vi "Initialize With IDN.vi"(0 "VISA resource name":refnum<visa-resource-name>="GPIB0::16::INSTR", 9 "Serial Configuration":T1={"Baud Rate (9600)"=19200, "Flow Control (1: XON/XOFF)"=1, "Termination Char (0:CR)"=0} {"Termination Char (0:CR)" items=["CR", "LF"]; "Flow Control (1: XON/XOFF)" items=["None", "XON/XOFF", "RTS/CTS (2701 Only)", "XON/XOFF & RTS/CTS (2701 Only)"]; "Baud Rate (9600)" items=["300"=300, "600"=600, "1200"=1200, "2400"=2400, "4800"=4800, "9600"=9600, "19.2k"=19200, "38.4k (2701 Only)"=38400, "57.6k (2701 Only)"=57600, "115.2k (2701 Only)"=115200]}, 11 "error in (no error)":errorcluster) -> (4 "VISA resource name out":refnum<visa-resource-name>, 6 "ID Query read buffer":string, 15 "error out":errorcluster)   [LabVIEW 2015]
doc: "This VI opens a VISA session for the VISA resource name specified. You can optionally reset the instrument by setting the front panel reset control. You must run this VI before using any of the instrument driver VIs for this instrument.\n\nNotes:\n\n(1) This instrument driver supports serial communication. If problems are encountered when using serial communication, it is recommended to try using baud rates less than 19,200 and hardware handshaking. \n\n(2) If you do wish to use the serial interface, set the serial settings on the instrument to be the same as the serial settings on the block diagram and in Measurement & Automation Explorer.\n\n(3) This VI sets the instrument to *RST conditions as listed in the manual. This does not include clearing the buffer."
uses:
  <instrlib>/Keithley 27XX/Keithley 27XX.lvlib
panel:
  # "© 2005 National Instruments Corporation.  ALL RIGHTS RESERVED."
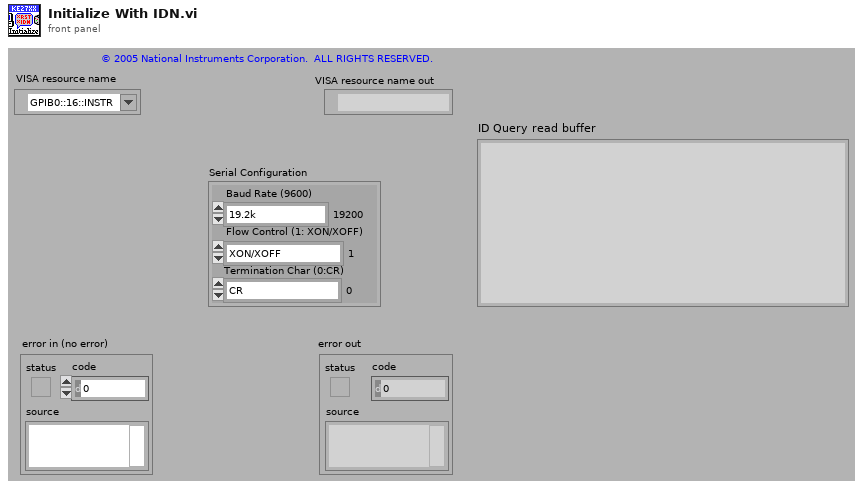
[diagram p1: front panel]
types:
  T1 = cluster{"Baud Rate (9600)":u32, "Flow Control (1: XON/XOFF)":u16, "Termination Char (0:CR)":u16}
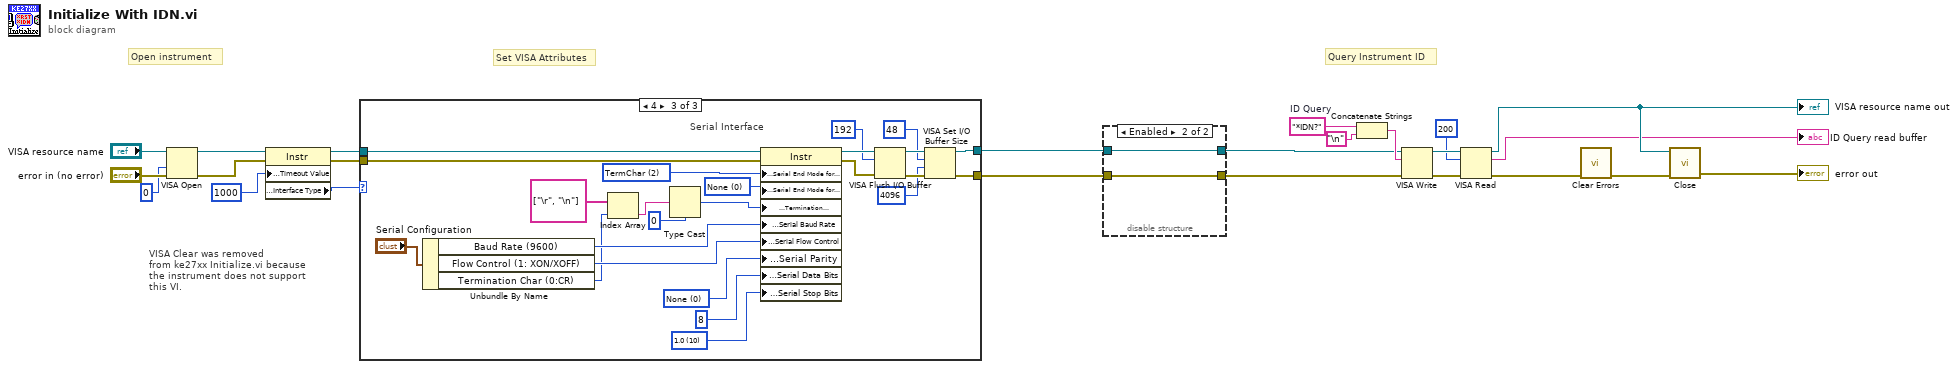
[diagram p0: block diagram]
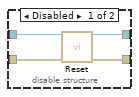
[diagram p2: hidden frame]
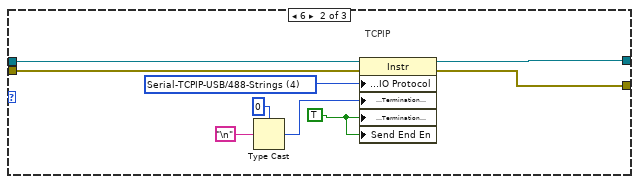
[diagram p4: hidden frame]
diagram:
  w8 = "*IDN?"  # ID Query
  # "VISA Clear was removed\nfrom ke27xx Initialize.vi because \nthe instrument does not support\nthis VI."
  # "Set VISA Attributes"
  # "Query Instrument ID"
  # "Open instrument"
  n1 = VISA Open(access mode=u32 0, error in (no error)="error in (no error)", VISA resource name="VISA resource name") -> (VISA resource name=w14:refnum<visa-resource-name>, error out=w15:errorcluster)  [unwired: 2 in]
  n2 = property class="Instr"(reference=w14, error in=w15, "General Settings:Timeout Value"=u32 1000) -> (reference out=w23:refnum<visa-resource-name>, error out=w24:errorcluster, "Interface Information:Interface Type"=w18:u16)
  n3 = case shown="4" w18 {
    tunnel: [w25 w32 w56] -> w2
    tunnel: [w26 w31 w53] -> w3
    tunnel: w23 -> [w25 w35 w58]
    tunnel: w24 -> [w26 w33 w59]
    frame 1, Default {
      # "GPIB"
    }
    frame 6 {
      w34 = u16 4 items=["Normal"=1, "VXI/FDC"=2, "GPIB/HS488"=3, "Serial-TCPIP-USB/488-Strings"=4, "USBTMC/Vendor-Specific"=5] ("Message Based Settings:IO Protocol")
      w27 = TRUE ("Message Based Settings:Termination Character Enable")
      # "TCPIP"
      n4 = Type Cast(type=u8 0, x="\n") -> (*(type *) &x=w28:u8)
      n5 = property class="Instr"(reference=w35, error in=w33, "Message Based Settings:IO Protocol"=w34, "Message Based Settings:Termination Character"=w28, "Message Based Settings:Termination Character Enable"=w27, "Send End En"=w27) -> (reference out=w32:refnum<visa-resource-name>, error out=w31:errorcluster)
    }
    frame 4 {
      w39 = u16 0 items=["None", "LastBit", "TermChar", "Break"] ("Serial Settings:Serial End Mode for Writes")
      w40 = u16 10 items=["1.0"=10, "1.5"=15, "2.0"=20] ("Serial Settings:Serial Stop Bits")
      w42 = u16 0 items=["None", "Odd", "Even", "Mark", "Space"] ("Serial Settings:Serial Parity")
      w43 = u16 2 items=["None", "LastBit", "TermChar"] ("Serial Settings:Serial End Mode for Reads")
      # "Serial Interface"
      n6 = Unbundle By Name("Serial Configuration") -> ("Baud Rate (9600)"=w45:u32, "Flow Control (1: XON/XOFF)"=w44:u16, "Termination Char (0:CR)"=w36:u16)
      n7 = Index Array(array=string[] ["\r", "\n"], index=w36) -> (element=w38:string)
      n8 = Type Cast(type=u8 0, x=w38) -> (*(type *) &x=w47:u8)
      n9 = property class="Instr"(reference=w58, error in=w59, "Serial Settings:Serial End Mode for Reads"=w43, "Serial Settings:Serial End Mode for Writes"=w39, "Message Based Settings:Termination Character"=w47, "Serial Settings:Serial Baud Rate"=w45, "Serial Settings:Serial Flow Control"=w44, "Serial Settings:Serial Parity"=w42, "Serial Settings:Serial Data Bits"=u16 8, "Serial Settings:Serial Stop Bits"=w40) -> (reference out=w52:refnum<visa-resource-name>, error out=w55:errorcluster)
      n10 = VISA Flush I/O Buffer(VISA resource name=w52, mask (16)=u16 192, error in (no error)=w55) -> (VISA resource name out=w57:refnum<visa-resource-name>, error out=w54:errorcluster)
      n11 = VISA Set I/O Buffer Size(VISA resource name=w57, mask (16)=u16 48, size (4096)=u32 4096 ("size (0)"), error in (no error)=w54) -> (VISA resource name out=w56:refnum<visa-resource-name>, error out=w53:errorcluster)
    }
  }
  n12 = disable-structure shown="Enabled" {
    disable-tunnel: [w63 w65] -> w5
    disable-tunnel: [w62 w64] -> w4
    disable-tunnel: w3 -> [w61 w64]
    disable-tunnel: w2 -> [w60 w65]
    frame Disabled {
      n13 = call <instrlib>:"Reset.vi"("VISA resource name"=w60, "error in (no error)"=w61) -> ("VISA resource name out"=w63:refnum<visa-resource-name>, "error out"=w62:errorcluster)  [unwired: 12 in]
    }
    frame Enabled {
    }
  }
  n14 = Concatenate Strings(w8, "\n") -> (w6:string)
  n15 = VISA Write(VISA resource name=w5, write buffer=w6, error in (no error)=w4) -> (VISA resource name out=w13:refnum<visa-resource-name>, error out=w12:errorcluster)  [unwired: 1 out]
  n16 = VISA Read(VISA resource name=w13, byte count=u32 200, error in (no error)=w12) -> (VISA resource name out=w19:refnum<visa-resource-name>, read buffer=→"ID Query read buffer":string, error out=w11:errorcluster)  [unwired: 1 out]
  "VISA resource name out" <- w19
  n17 = call <vilib>:"Clear Errors.vi"("error in (no error)"=w11) -> ("error out"=w1:errorcluster)  [unwired: 5 in, 1 out]
  n18 = call <instrlib>:"Close.vi"("VISA resource name"=w19, "error in (no error)"=w1) -> ("error out"=→"error out":errorcluster)  [unwired: 13 in]
